vi "store unload Slot.vi"(6 "bufferLength":i32, 7 "slot":i32, 8 "error in (no error)":errorcluster, 9 "index":i32, 10 "result":cluster{"value":i32, "error":i32}, 11 "id":u32) -> (0 "error out":errorcluster, 1 "buffer":u8[](array[numeric]), 2 "result out":cluster{"value":i32, "error":i32}, 3 "id out":u32)   [LabVIEW 2021, in "BrainStem2_LabVIEW_Library.lvlib"]
doc: "aLIBEXPORT void __stdcall store_unloadSlot ( unsigned int* id, struct Result* result, const int index , const int slot, unsigned char * buffer, const int bufferLength ) ;"
uses:
  BrainStem2_LabVIEW_Library.lvlib
  BrainStem2_LabVIEW.dll
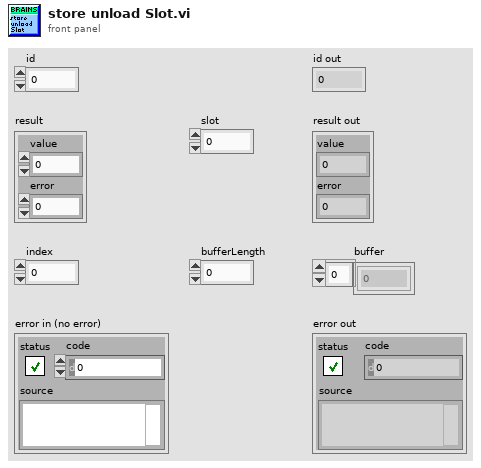
[diagram p1: front panel]
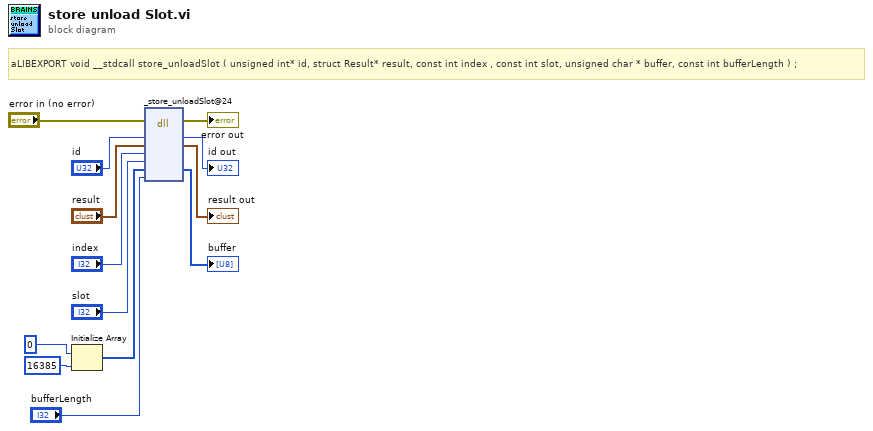
[diagram p0: block diagram]
diagram:
  # "aLIBEXPORT void __stdcall store_unloadSlot ( unsigned int* id, struct Result* result, const int index , const int slot, unsigned char * buffer, const int bufferLength ) ;"
  n1 = Initialize Array(u8 0 ("element"), 16385 ("dimension size")) -> (w7:u8[])
  n2 = dll-call lib="C:/DEV-TDS/Canary/T20029/T20029-80004 BS2 PROG SW/src/drivers/acroname/development/LabVIEW/BrainStem2_LabVIEW_w32/BrainStem2_LabVIEW_w32/BrainStem2_LabVIEW.*" fn="_store_unloadSlot@24"(error in="error in (no error)", "id"="id", "result"="result", "index"="index", "slot"="slot", "buffer"=w7, "bufferLength"="bufferLength") -> (error out=→"error out":errorcluster, "id"=→"id out":u32, "result"=→"result out":cluster{"value":i32, "error":i32}, "buffer"=→"buffer":u8[])  [unwired: 6 in, 1 out]
